vi "New Smoother 2.vi"(11 "GIC Input":T1={"     Use ?\nOff       On"=[FALSE, TRUE, FALSE, TRUE], "Mode:"=FALSE, "Rx Prop Port"="", "Hokuyo Port"="COM7", "Tx Prop  Port"="COM6", "Compass Port"="", "GPS Port"="", "Num of WPs"=0, "WP Lats and Longs"={"WP Lats"=[], "WP Longs"=[]}, "Obst Lats and Longs"={"Obst Lats"=[], "Obst Longs"=[]}, "Parameters"=[], "GPS Data"=[], "Compass"=0.0, "LMS Vector"=[], "Vision Vector"=[], "Direction Cmd"=0.0, "Speed Cmd"=0.0, "WP Vector"=[], "WP Number"=0, "Extra"=0, "SW Map"=[], "Path Cluster"={"Path x node"=[], "Path y node"=[]}} {"Obst Lats and Longs"."Obst Longs" format="%#_8g"; "Obst Lats and Longs"."Obst Lats" format="%#_8g"}) -> (3 "GIC Output":T1={"     Use ?\nOff       On"=[FALSE, TRUE, FALSE, TRUE], "Mode:"=FALSE, "Rx Prop Port"="", "Hokuyo Port"="COM7", "Tx Prop  Port"="COM6", "Compass Port"="", "GPS Port"="", "Num of WPs"=0, "WP Lats and Longs"={"WP Lats"=[], "WP Longs"=[]}, "Obst Lats and Longs"={"Obst Lats"=[], "Obst Longs"=[]}, "Parameters"=[], "GPS Data"=[], "Compass"=0.0, "LMS Vector"=[], "Vision Vector"=[], "Direction Cmd"=0.0, "Speed Cmd"=0.0, "WP Vector"=[], "WP Number"=0, "Extra"=0, "SW Map"=[], "Path Cluster"={"Path x node"=[], "Path y node"=[]}} {"Obst Lats and Longs"."Obst Longs" format="%#_8g"; "Obst Lats and Longs"."Obst Lats" format="%#_8g"})   [LabVIEW 2014]
panel:
  out "Hop Save":dbl
  out "Test 3":dbl
  out "Test 2":dbl
  in  "Path y test":dbl[](array[numeric])
  in  "Path x test":dbl[](array[numeric])
  in  "Test Parameters":dbl[](array[numeric])
  out "test 1":dbl
  # "New Smoother 2"
  # "Input:"
  # "Output"
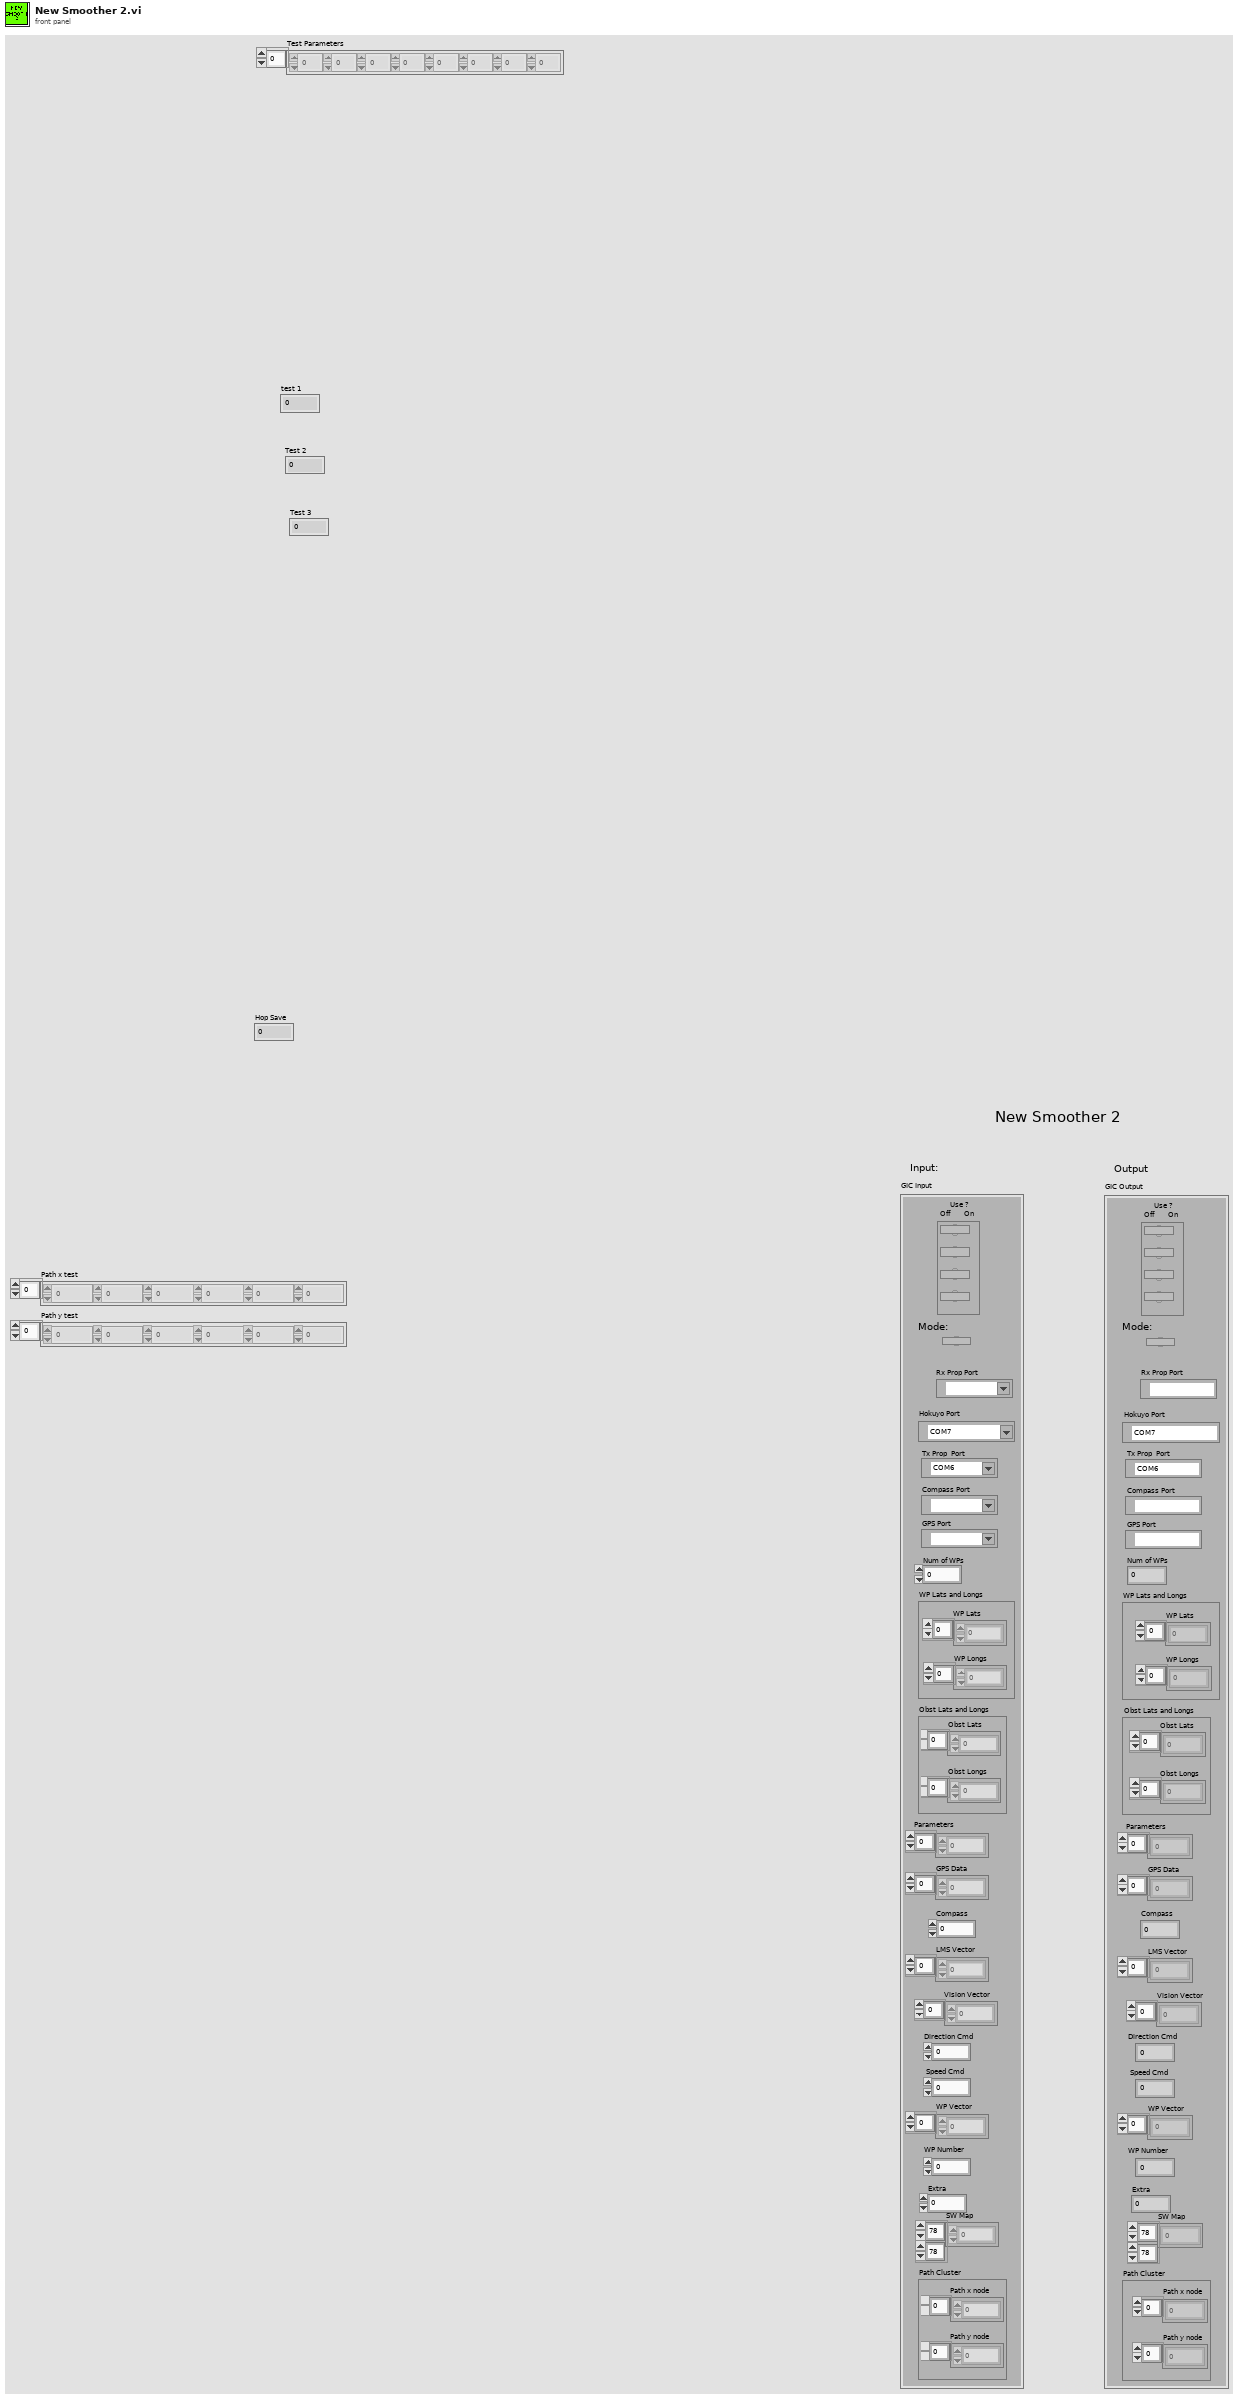
[diagram p1: front panel]
types:
  T1 = cluster{"     Use ?\nOff       On":bool[], "Mode:":bool, "Rx Prop Port":refnum<visa-resource-name>, "Hokuyo Port":refnum<visa-resource-name>, "Tx Prop  Port":refnum<visa-resource-name>, "Compass Port":refnum<visa-resource-name>, "GPS Port":refnum<visa-resource-name>, "Num of WPs":i16, "WP Lats and Longs":cluster{"WP Lats":dbl[], "WP Longs":dbl[]}, "Obst Lats and Longs":cluster{"Obst Lats":dbl[], "Obst Longs":dbl[]}, "Parameters":dbl[], "GPS Data":dbl[], "Compass":dbl, "LMS Vector":dbl[], "Vision Vector":dbl[], "Direction Cmd":dbl, "Speed Cmd":dbl, "WP Vector":dbl[], "WP Number":i32, "Extra":i16, "SW Map":i32[][], "Path Cluster":cluster{"Path x node":dbl[], "Path y node":dbl[]}}
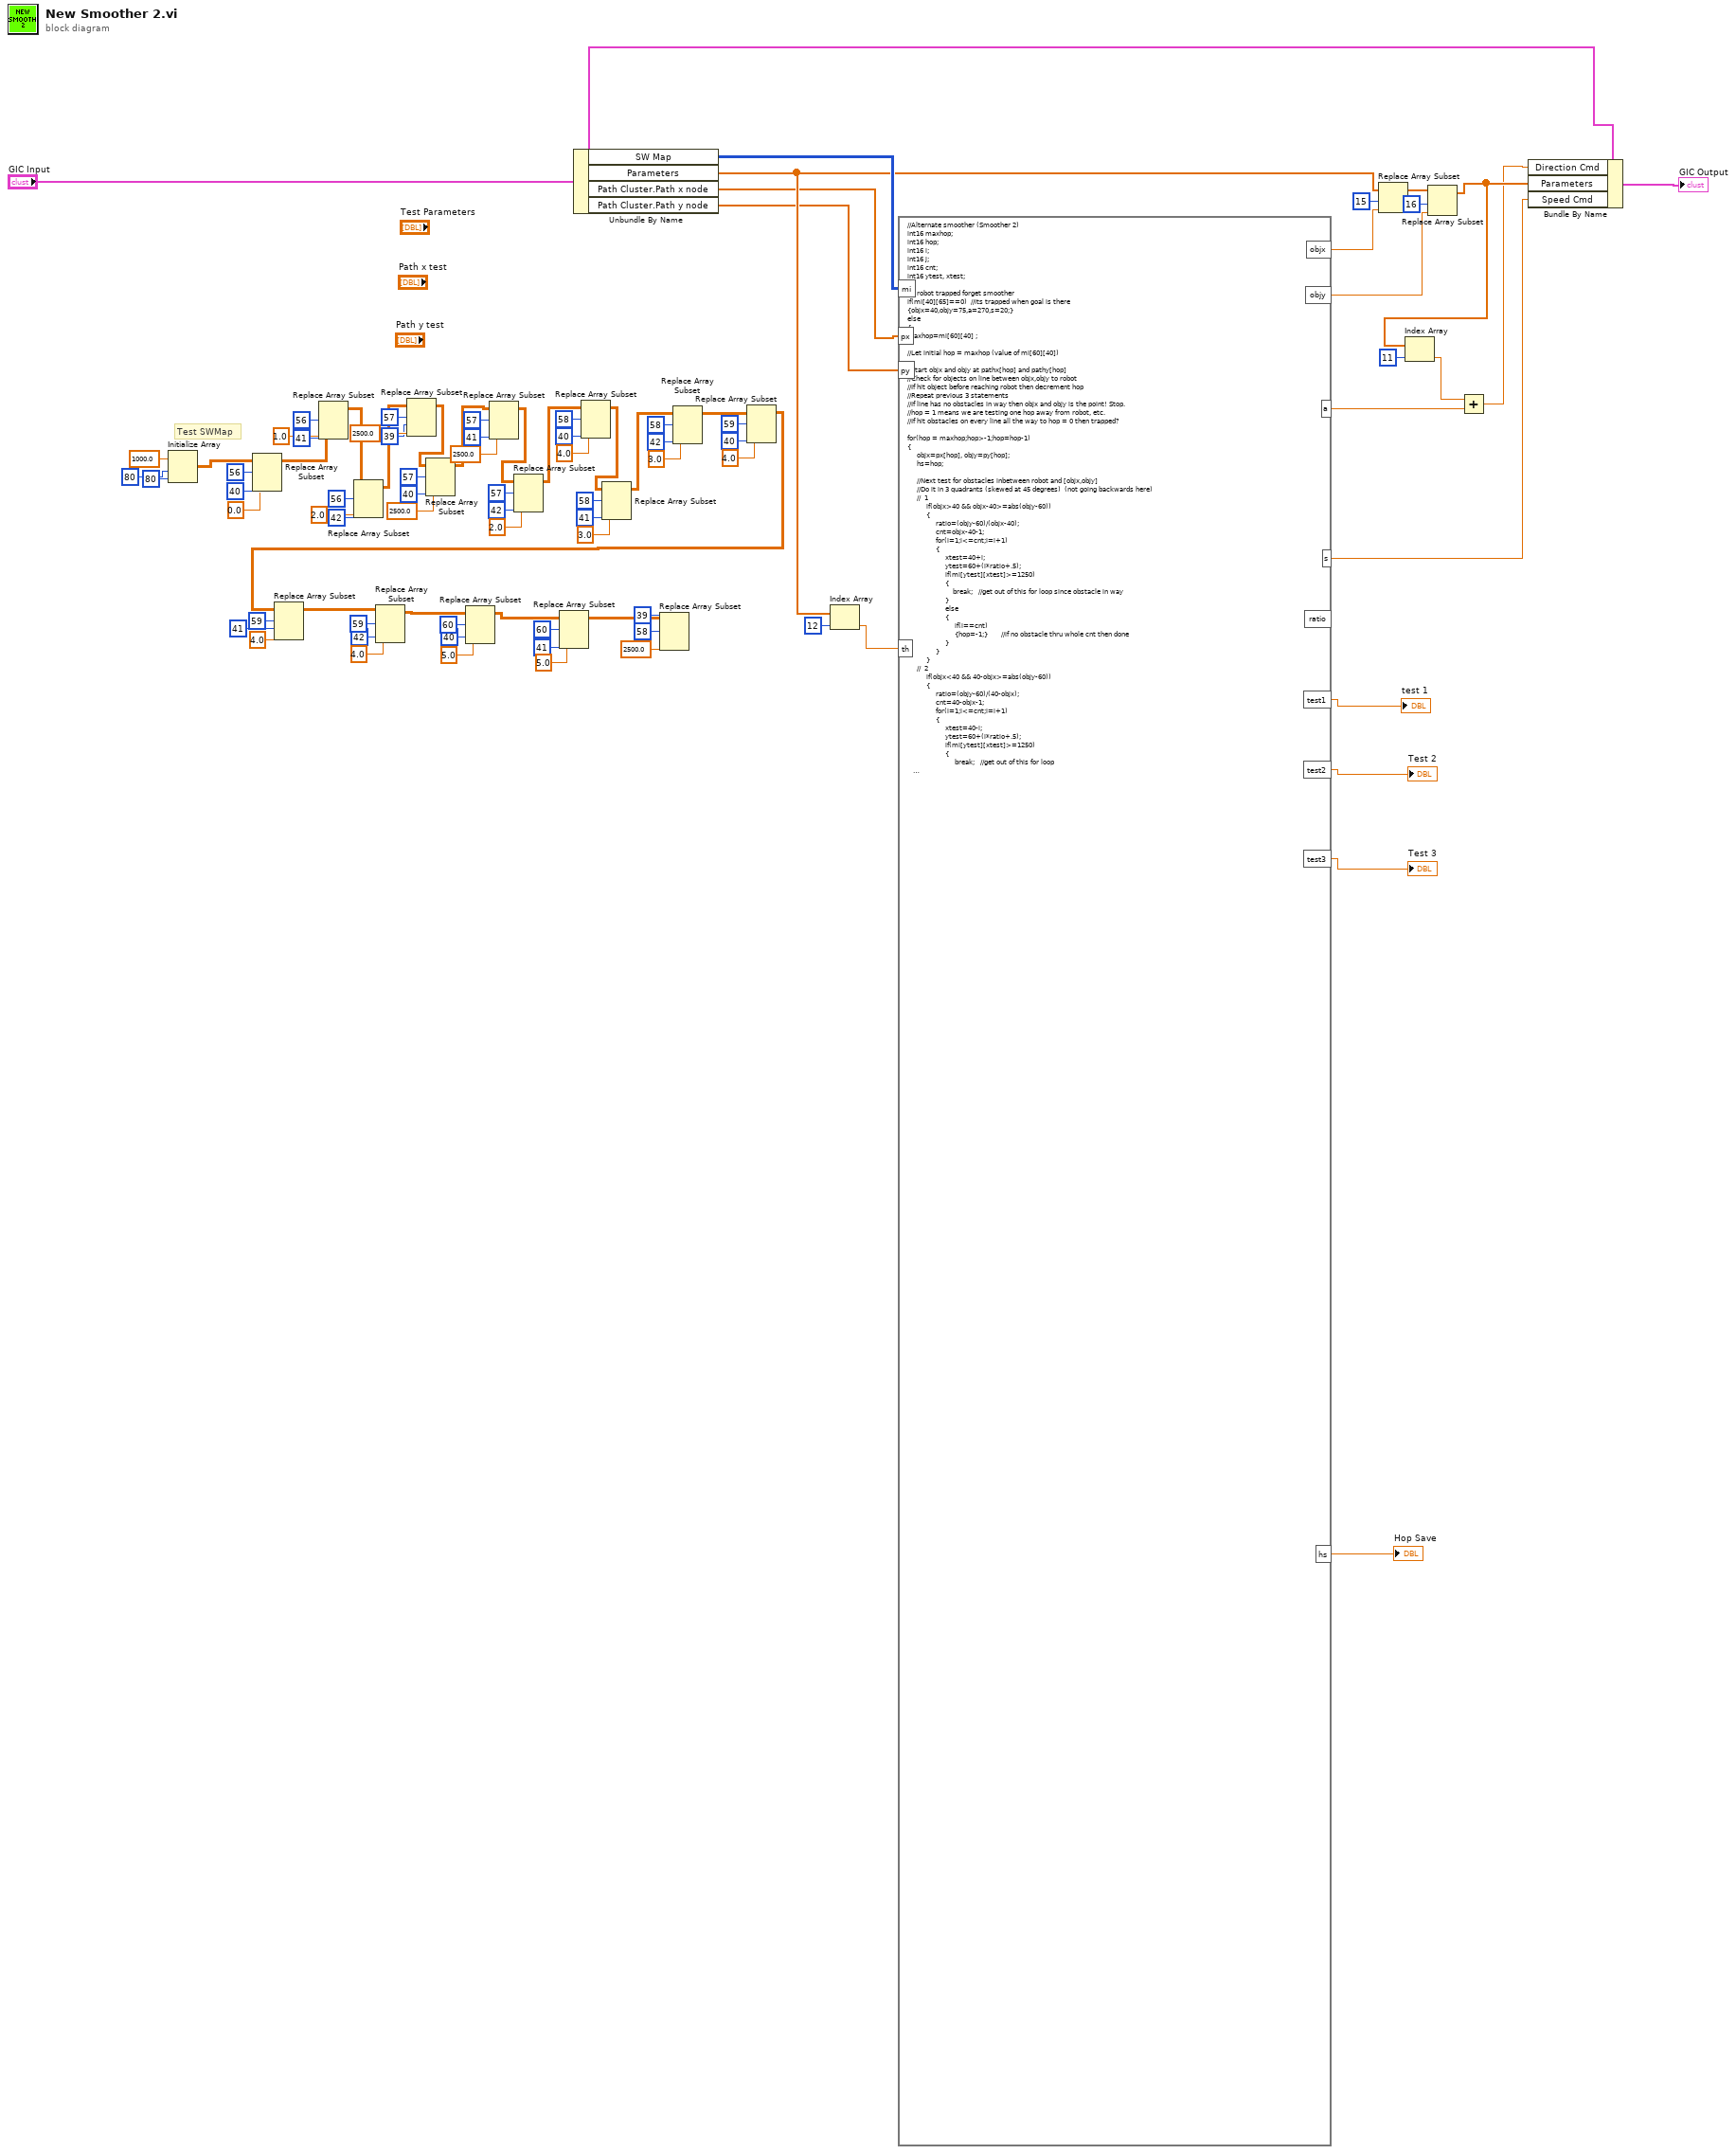
[diagram p0: block diagram]
diagram:
  # "Test SWMap"
  n1 = Initialize Array(1000.0 ("element"), 80 ("dimension size"), 80 ("dimension size")) -> (w87:dbl[][])
  n2 = Replace Array Subset(array=w87, new element=0.0 ("new element/subarray"), index (row)=56, index (col)=40 ("disabled index (col)")) -> (w83:dbl[][])
  n3 = Replace Array Subset(array=w83, new element=1.0 ("new element/subarray"), index (row)=56, index (col)=41 ("disabled index (col)")) -> (w79:dbl[][])
  n4 = Replace Array Subset(array=w79, new element=2.0 ("new element/subarray"), index (row)=56, index (col)=42 ("disabled index (col)")) -> (w74:dbl[][])
  n5 = Replace Array Subset(array=w74, new element=2500.0 ("new element/subarray"), index (row)=57, index (col)=39 ("disabled index (col)")) -> (w70:dbl[][])
  n6 = Replace Array Subset(array=w70, new element=2500.0 ("new element/subarray"), index (row)=57, index (col)=40 ("disabled index (col)")) -> (w66:dbl[][])
  n7 = Replace Array Subset(array=w66, new element=2500.0 ("new element/subarray"), index (row)=57, index (col)=41 ("disabled index (col)")) -> (w62:dbl[][])
  n8 = Replace Array Subset(array=w62, new element=2.0 ("new element/subarray"), index (row)=57, index (col)=42 ("disabled index (col)")) -> (w58:dbl[][])
  n9 = Unbundle By Name("GIC Input") -> ("SW Map"=w21:i32[][], "Parameters"=w8:dbl[], "Path Cluster.Path x node"=w2:dbl[], "Path Cluster.Path y node"=w1:dbl[])
  n10 = Replace Array Subset(array=w58, new element=4.0 ("new element/subarray"), index (row)=58, index (col)=40 ("disabled index (col)")) -> (w54:dbl[][])
  n11 = Replace Array Subset(array=w54, new element=3.0 ("new element/subarray"), index (row)=58, index (col)=41 ("disabled index (col)")) -> (w50:dbl[][])
  n12 = Replace Array Subset(array=w50, new element=3.0 ("new element/subarray"), index (row)=58, index (col)=42 ("disabled index (col)")) -> (w46:dbl[][])
  n13 = Replace Array Subset(array=w46, new element=4.0 ("new element/subarray"), index (row)=59, index (col)=40 ("disabled index (col)")) -> (w42:dbl[][])
  n14 = Replace Array Subset(array=w42, new element=4.0 ("new element/subarray"), index (row)=59, index (col)=41 ("disabled index (col)")) -> (w41:dbl[][])
  n15 = Replace Array Subset(array=w41, new element=4.0 ("new element/subarray"), index (row)=59, index (col)=42 ("disabled index (col)")) -> (w40:dbl[][])
  n16 = Replace Array Subset(array=w40, new element=5.0 ("new element/subarray"), index (row)=60, index (col)=40 ("disabled index (col)")) -> (w39:dbl[][])
  n17 = Replace Array Subset(array=w39, new element=5.0 ("new element/subarray"), index (row)=60, index (col)=41 ("disabled index (col)")) -> (w38:dbl[][])
  n18 = Replace Array Subset(array=w38, new element=2500.0 ("new element/subarray"), index (row)=58, index (col)=39 ("disabled index (col)")) -> ()  [unwired: 1 out]
  n19 = Index Array(array=w8, index=12) -> (element=w6:dbl)
  n20 = formula code="//Alternate smoother (Smoother 2)\nint16 maxhop;\nint16 hop;\nint16 i;\nint16 j;\nint16 cnt;\nint16 ytest, xtest;\n\n//If robot trapped forget smoother\nif(mi[40][65]==0)  //its trapped when goal is there\n{objx=40,objy=75,a=270,s=20;}\nelse\n{\nmaxhop=mi[60][40] ;\n\n//Let initial hop = maxhop (value of mi[60][40])\n\n//Start objx and objy at pathx[hop] and pathy[hop]\n//Check for objects on line between objx,objy to robot\n//If hit object before reaching robot then decrement hop\n//Repeat previous 3 statements\n//If line has no obstacles in way then objx and objy is the point! Stop.\n//hop = 1 means we are testing one hop away from robot, etc.\n//If hit obstacles on every line all the way to hop = 0 then trapped?\n\nfor(hop = maxhop;hop>-1;hop=hop-1)\n{\n     objx=px[hop], objy=py[hop];\n     hs=hop;\n      \n     //Next test for obstacles inbetween robot and [objx,objy]\n     //Do it in 3 quadrants (skewed at 45 degrees)  (not going backwards here)\n     //  1\n          if(objx>40 && objx-40>=abs(objy-60))\n          {\n               ratio=(objy-60)/(objx-40);\n               cnt=objx-40-1;\n               for(i=1;i<=cnt;i=i+1)\n               {\n                    xtest=40+i;\n                    ytest=60+(i*ratio+.5);\n                    if(mi[ytest][xtest]>=1250)\n                    {\n                        break;   //get out of this for loop since obstacle in way\n                    }\n                    else\n                    {\n                         if(i==cnt)\n                         {hop=-1;}       //if no obstacle thru whole cnt then done\n                    }\n               }\n          }\n     //  2\n          if(objx<40 && 40-objx>=abs(objy-60))\n          {\n               ratio=(objy-60)/(40-objx);\n               cnt=40-objx-1;\n               for(i=1;i<=cnt;i=i+1)\n               {\n                    xtest=40-i;\n                    ytest=60+(i*ratio+.5);\n                    if(mi[ytest][xtest]>=1250)\n                    {\n                         break;   //get out of this for loop\n                    }\n                    else\n                    {\n                         if(i==cnt)\n                         {hop=-1;}       //if no obstacle thru whole cnt then done\n                    }\n               }\n          }\n          //   3\n               if(objy<60 && 60-objy>=abs(objx-40))\n               {\n                    ratio=(objx-40)/(60-objy);\n                    cnt=60-objy-1;\n                    for(j=1;j<=cnt;j=j+1)\n                    {\n                         ytest=60-j;\n                         xtest=40+(j*ratio+.5);\n                         if(mi[ytest][xtest]>=1250)\n                         {\n                              break;   //get out of this for loop\n                         }\n                         else\n                         {\n                              if(j==cnt)\n                              {hop=-1;}       //if no obstacle thru whole cnt then done\n                         }\n                    }\n               }\n}\n\n//Next calculate angle based on robot to [objx,objy]\n//0 degrees is on right and 180 on left, 90 is straight ahead\n//1st Quadrant\n     if(objx>40)\n     {\n          if(objy<60)\n               {a=atan((60-objy)/(objx-40))*180/3.14159;}\n          else if(objy>60)  //if objy is behind robot, just go back (trapped)\n               {a=270;}\n          else\n               {a=0;}   //go right if objy = 60 and objx >40\n     }\n//2nd Quadrant\n     if(objx<40)\n     {\n          if(objy<60)\n               {a=180+atan((60-objy)/(objx-40))*180/3.14159;}\n          else if(objy>60)  //if objy is behind robot, just go back (trapped)\n               {a=270;}\n          else\n               {a=180;}   //go left if objy = 60 and objx <40\n     }\n//If objx and objy point is straight ahead\n     if(objx==40 && objy<60)\n          {a=90;}\n//if objx and oby on robot then trapped\n     if(objx==40 && objy==60)\n          {a=270;}\n//Next calculate speed based on distance of [objx,objy] from robot\n     s=abs(40-objx)+abs(60-objy);  //max of 100 if head for far corner\n//Limit minimum speed\n     //if(s<60)\n     //     {s = 60;}\n//Speed warp\n     if(s>0)\n          {\n               if(s<=th)\n                    {s=th;}\n          }\n//end of else for when robot is not trapped\n\n//test1=objx;\n//test2=objy;\n//test3=hop;\n} //end of big if to check if robot trapped"("mi"=w21, "px"=w2, "py"=w1, "th"=w6) -> ("test1"=→"test 1":dbl, "objx"=w17:dbl, "objy"=w14:dbl, "a"=w10:dbl, "s"=w19:dbl, "test2"=→"Test 2":dbl, "test3"=→"Test 3":dbl, "hs"=→"Hop Save":dbl)  [unwired: 1 out]
  n21 = Replace Array Subset(array=w8, new element=w17, index=15) -> (w16:dbl[])
  n22 = Replace Array Subset(array=w16, new element=w14, index=16) -> (w13:dbl[])
  n23 = Index Array(array=w13, index=11) -> (element=w11:dbl)
  n24 = Add(x=w11, y=w10) -> (x+y=w9:dbl)
  n25 = Bundle By Name(cluster="GIC Input", "Direction Cmd"=w9, "Parameters"=w13, "Speed Cmd"=w19) -> (→"GIC Output":T1)
